vi "Up_Draw+.vi"(6 "Color":u32(colorbox)=16711680, 7 "y":dbl=20.0 format="%#_13g", 10 "Center":cluster{"x":dbl, "y":dbl}, 11 "Image":T1) -> (3 "Image Out":T1)   [LabVIEW 2019]
uses:
  <vilib>/vision/Image Controls.llb/IMAQ Image.ctl
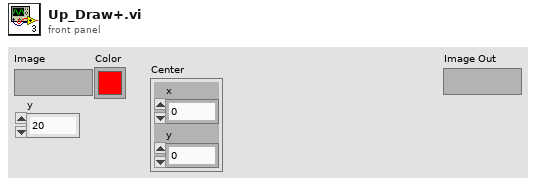
[diagram p1: front panel]
types:
  T1 = typedef "IMAQ Image.ctl" = refnum<image>
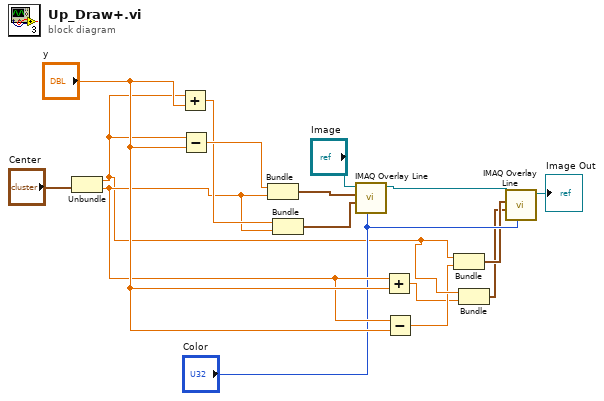
[diagram p0: block diagram]
diagram:
  n1 = Unbundle("Center") -> ("x"=w6:dbl, "y"=w11:dbl)
  n2 = Add(x=w6, y="y") -> (x+y=w12:dbl)
  n3 = Subtract(x=w6, y="y") -> (x-y=w13:dbl)
  n4 = Bundle(w13, "y"=w11) -> (w14:cluster{dbl, "y":dbl})  [unwired: 1 in]
  n5 = Bundle(w12, "y"=w11) -> (w10:cluster{dbl, "y":dbl})  [unwired: 1 in]
  n6 = call "IMAQ Overlay Line"("Color"="Color", "End Point"=w10, "Start Point"=w14, "Image"="Image") -> ("Image Out"=w8:T1)  [unwired: 6 in, 1 out]
  n7 = Add(x=w11, y="y") -> (x+y=w4:dbl)
  n8 = Subtract(x=w11, y="y") -> (x-y=w5:dbl)
  n9 = Bundle("x"=w6, w5) -> (w3:cluster{"x":dbl, dbl})  [unwired: 1 in]
  n10 = Bundle("x"=w6, w4) -> (w2:cluster{"x":dbl, dbl})  [unwired: 1 in]
  n11 = call "IMAQ Overlay Line"("Color"="Color", "End Point"=w2, "Start Point"=w3, "Image"=w8) -> ("Image Out"=→"Image Out":T1)  [unwired: 6 in, 1 out]
